vi "曲线模型计算.vi"(11 "曲线模型":T2={"标液浓度1"=0.0, "测量吸光度1"=0.0, "样品1启用"=FALSE, "标液浓度2"=0.0, "测量吸光度2"=0.0, "样品2启用"=FALSE, "标液浓度3"=0.0, "测量吸光度3"=0.0, "样品3启用"=FALSE, "标液浓度4"=0.0, "测量吸光度4"=0.0, "样品4启用"=FALSE, "标液浓度5"=0.0, "测量吸光度5"=0.0, "样品5启用"=FALSE, "模型"=enum."线性", "精度"=4.0, "XY图"=[], "拟合公式"="", "r^2"=0.0, "标样一校准时间"=timestamp(0 s since 1904-01-01), "标样二校准时间"=timestamp(0 s since 1904-01-01), "标样三校准时间"=timestamp(0 s since 1904-01-01), "标样四校准时间"=timestamp(0 s since 1904-01-01), "标样五校准时间"=timestamp(0 s since 1904-01-01), "二次方程"={"x^2"=0.0, "K"=0.0, "B"=0.0}, "标定时间"=timestamp(0 s since 1904-01-01), "拟合公式 2"="", "r^2 2"=0.0} {"r^2 2" format="%.7f"; "标定时间" format="%<%Y/%m/%d %H:%M:%S>T"; "标样五校准时间" format="%<%Y/%m/%d %H:%M:%S>T"; "标样四校准时间" format="%<%Y/%m/%d %H:%M:%S>T"; "标样三校准时间" format="%<%Y/%m/%d %H:%M:%S>T"; "标样二校准时间" format="%<%Y/%m/%d %H:%M:%S>T"; "标样一校准时间" format="%<%Y/%m/%d %H:%M:%S>T"; "r^2" format="%.7f"; "测量吸光度5" format="%#.6f"; "测量吸光度4" format="%#.6f"; "测量吸光度3" format="%#.6f"; "测量吸光度2" format="%#.6f"; "测量吸光度1" format="%#.6f"}) -> (1 "公式切换阈值滴定数(0~9999)":dbl, 2 "二次方程 2":cluster{"x^2":dbl, "K":dbl, "B":dbl}, 3 "输出簇":T1)   [LabVIEW 2016, in "斯坦道CODMn新电路板.lvlib"]
uses:
  <vilib>/Analysis/6fits.llb/Curve Fitting Criteria.ctl
  <vilib>/Analysis/NI_AALPro.lvlib
panel:
  # "校准时间"
  # "标液浓度"
  # "滴定数"
  # "标液一"
  # "标液二"
  # "标液三"
  # "零点"
  # "跨度"
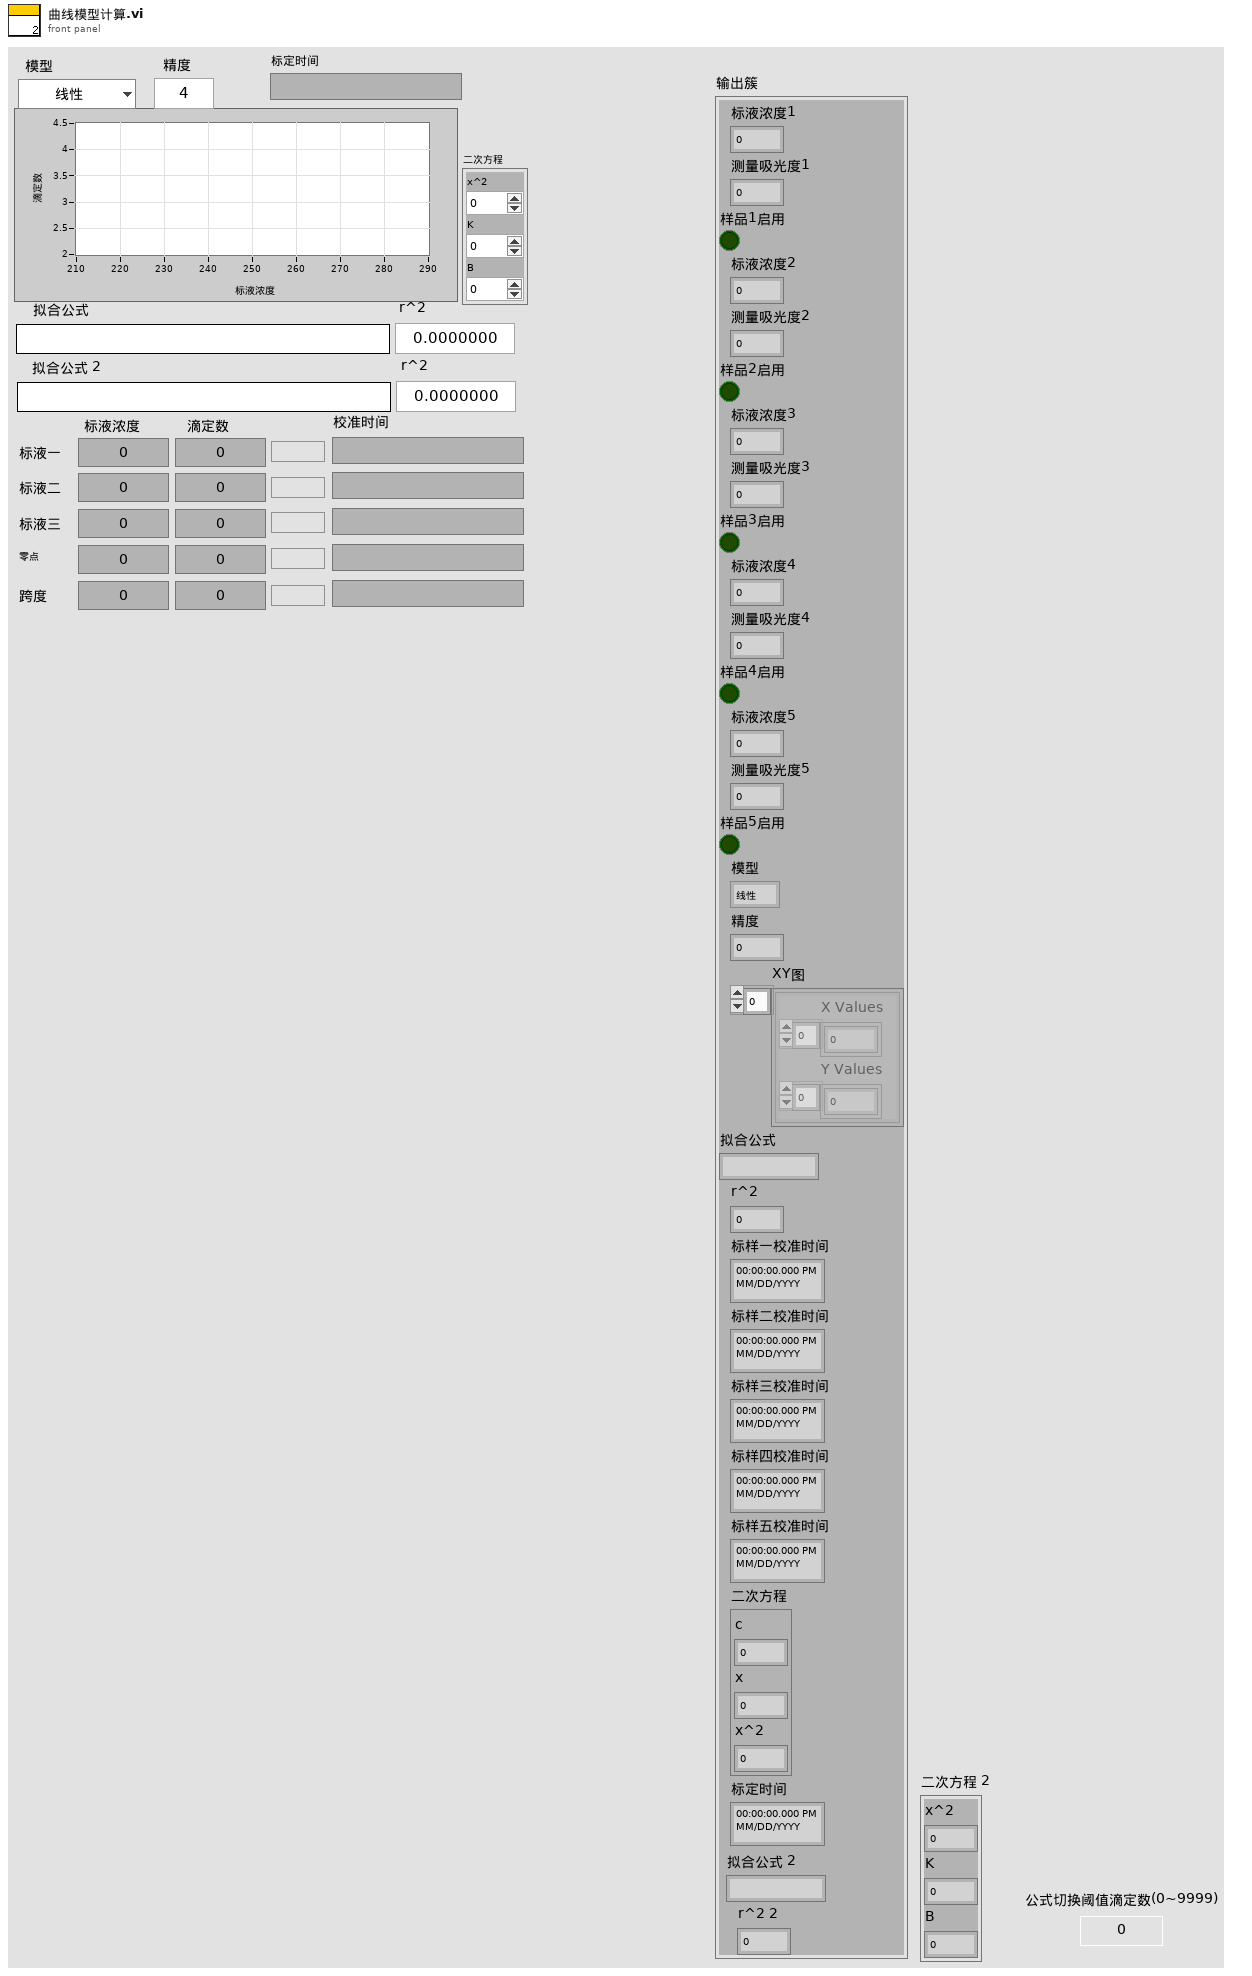
[diagram p1: front panel]
types:
  T1 = cluster{"标液浓度1":dbl, "测量吸光度1":dbl, "样品1启用":bool, "标液浓度2":dbl, "测量吸光度2":dbl, "样品2启用":bool, "标液浓度3":dbl, "测量吸光度3":dbl, "样品3启用":bool, "标液浓度4":dbl, "测量吸光度4":dbl, "样品4启用":bool, "标液浓度5":dbl, "测量吸光度5":dbl, "样品5启用":bool, "模型":enum32{"线性", "多项式", "折线"}, "精度":dbl, "XY图":cluster{"X Values":dbl[], "Y Values":dbl[]}[], "拟合公式":string, "r^2":dbl, "标样一校准时间":timestamp, "标样二校准时间":timestamp, "标样三校准时间":timestamp, "标样四校准时间":timestamp, "标样五校准时间":timestamp, "二次方程":cluster{"c":dbl, "x":dbl, "x^2":dbl}, "标定时间":timestamp, "拟合公式 2":string, "r^2 2":dbl}
  T2 = cluster{"标液浓度1":dbl, "测量吸光度1":dbl, "样品1启用":bool, "标液浓度2":dbl, "测量吸光度2":dbl, "样品2启用":bool, "标液浓度3":dbl, "测量吸光度3":dbl, "样品3启用":bool, "标液浓度4":dbl, "测量吸光度4":dbl, "样品4启用":bool, "标液浓度5":dbl, "测量吸光度5":dbl, "样品5启用":bool, "模型":enum32{"线性", "多项式", "折线"}, "精度":dbl, "XY图":cluster{"X Values":dbl[], "Y Values":dbl[]}[], "拟合公式":string, "r^2":dbl, "标样一校准时间":timestamp, "标样二校准时间":timestamp, "标样三校准时间":timestamp, "标样四校准时间":timestamp, "标样五校准时间":timestamp, "二次方程":cluster{"x^2":dbl, "K":dbl, "B":dbl}, "标定时间":timestamp, "拟合公式 2":string, "r^2 2":dbl}
  T3 = typedef "NI_AALPro.lvlib/Curve Fitting Criteria.ctl" = u16
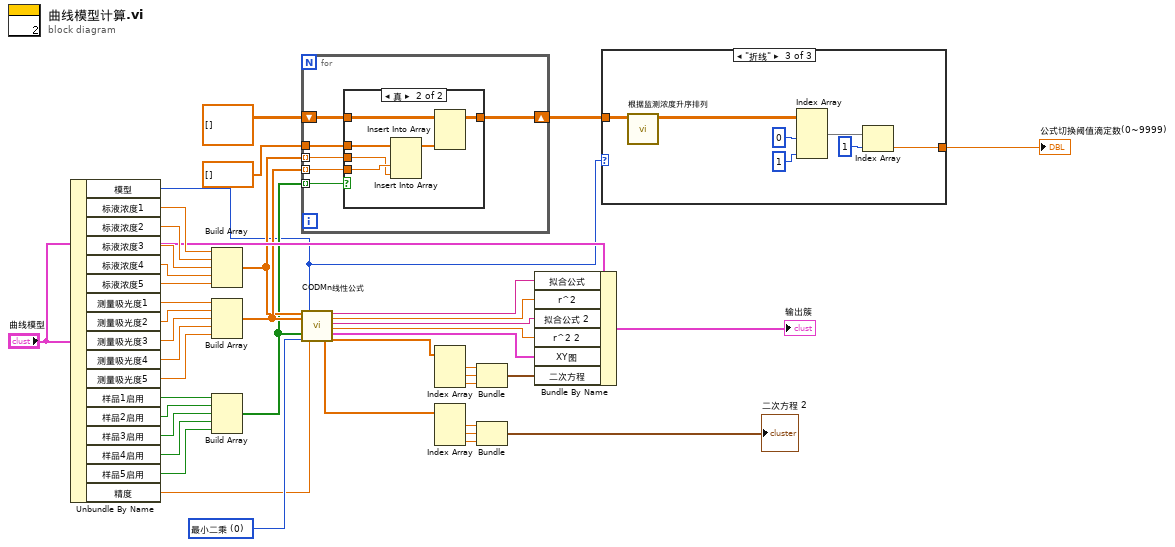
[diagram p0: block diagram]
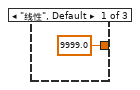
[diagram p2: hidden frame]
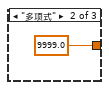
[diagram p3: hidden frame]
diagram:
  w27 = T3 0 items=["最小二乘", "最小绝对残差", "Bisquare"] ("method")
  n1 = Unbundle By Name("曲线模型") -> ("模型"=w1:enum32{"线性", "多项式", "折线"}, "标液浓度1"=w42:dbl, "标液浓度2"=w41:dbl, "标液浓度3"=w40:dbl, "标液浓度4"=w39:dbl, "标液浓度5"=w38:dbl, "测量吸光度1"=w37:dbl, "测量吸光度2"=w36:dbl, "测量吸光度3"=w35:dbl, "测量吸光度4"=w34:dbl, "测量吸光度5"=w33:dbl, "样品1启用"=w32:bool, "样品2启用"=w31:bool, "样品3启用"=w30:bool, "样品4启用"=w29:bool, "样品5启用"=w28:bool, "精度"=w26:dbl)
  n2 = Build Array(w42, w41, w40, w39, w38) -> (w4:dbl[])
  n3 = Build Array(w37, w36, w35, w34, w33) -> (w5:dbl[])
  n4 = Build Array(w32, w31, w30, w29, w28) -> (w3:bool[])
  n5 = for {
    tunnel: w3 -> [w43] mode=indexing
    tunnel: w5 -> [w46] mode=indexing
    tunnel: w4 -> [w45] mode=indexing
    shift-right: [w44] -> w6
    shift-left: dbl[][] [] ("标液浓度") -> [w48]
    tunnel: dbl[] [] ("监测浓度") -> [w47]
    n6 = case shown="真" w43 {
      tunnel: w48 -> [w49 w55]
      tunnel: w47 -> [_ w54]
      tunnel: w46 -> [_ w53]
      tunnel: w45 -> [_ w52]
      tunnel: [w49 w50] -> w44
      frame False {
      }
      frame True {
        n7 = Insert Into Array(array=w54, new element #1=w53, new element #2=w52) -> (w51:dbl[])  [unwired: 1 in]
        n8 = Insert Into Array(array=w55, new element=w51) -> (w50:dbl[][])  [unwired: 2 in]
      }
    }
  }
  n9 = call "CODMn线性公式.vi"("标液浓度"=w4, "信号值"=w5, "启用"=w3, "method"=w27, "模型"=w1, "精度"=w26) -> ("Polynomial Coefficients 2"=w12:dbl[], "拟合方程"=w25:string, "r^2"=w24:dbl, "拟合方程 2"=w23:string, "r^2 2"=w22:dbl, "XY图"=w21:cluster{"X Values":dbl[], "Y Values":dbl[]}[], "Polynomial Coefficients"=w17:dbl[])  [unwired: 7 in]
  n10 = Index Array(array=w17) -> (element #1=w20:dbl, element #2=w19:dbl, element #3=w18:dbl)  [unwired: 3 in]
  n11 = Index Array(array=w12) -> (element #1=w13:dbl, element #2=w14:dbl, element #3=w15:dbl)  [unwired: 3 in]
  n12 = Bundle("数值"=w20, "数值"=w19, "数值"=w18) -> (w16:cluster{"数值":dbl, "数值":dbl, "数值":dbl})  [unwired: 1 in]
  n13 = Bundle("数值"=w13, "数值"=w14, "数值"=w15) -> (→"二次方程 2":cluster{"数值":dbl, "数值":dbl, "数值":dbl})  [unwired: 1 in]
  n14 = Bundle By Name(cluster="曲线模型", "拟合公式"=w25, "r^2"=w24, "拟合公式 2"=w23, "r^2 2"=w22, "XY图"=w21, "二次方程"=w16) -> (→"输出簇":T2)
  n15 = case shown="\"折线\"" w1 {
    tunnel: w6 -> [_ _ w64]
    tunnel: [9999.0 ("数值") 9999.0 ("数值") w58] -> w2
    frame "线性", Default {
    }
    frame "多项式" {
    }
    frame "折线" {
      n16 = call "根据监测浓度升序排列.vi"("标液浓度输入"=w64) -> ("输出数组"=w61:dbl[][])  [unwired: 10 in]
      n17 = Index Array(array=w61, index (col) #1=0 ("禁用的索引 (列)"), index (col) #2=1 ("索引 (列)")) -> (element #1=w59:dbl[])  [unwired: 2 in, 1 out]
      n18 = Index Array(array=w59, index=1 ("索引")) -> (element=w58:dbl)
    }
  }
  "公式切换阈值滴定数(0~9999)" <- w2
